vi "Measurement Logic.vi"(8 "error in":errorcluster, 11 "Measurement Configuration":T3={"Load Current in A"=0.005, "Nominal Output Voltage in V"=3.3, "Start"=4.0, "Stop"=6.0, "Step"=0.1, "Input SMU"="", "Load SMU"="", "Input DMM"="", "Load DMM"=""} {"Start" format="%#_13g"; "Nominal Output Voltage in V" format="%#_13g"; "Load Current in A" format="%#_13g"}) -> (0 "error out":errorcluster, 3 "Measurement Results":T2)   [LabVIEW 2020, in "LineRegulation.lvlib"]
uses:
  LineRegulation.lvlib
  Measurement Configuration.ctl
  Measurement Results.ctl
  Reusables/TestResults.ctl
  Reusables/TestInputs.ctl
  Reusables/Advanced Settings.ctl
  Reusables/Prepare Fn Configurations.ctl
  Reusables/Load Output Function.ctl
  Reusables/Stimulus And Measure.ctl
  67fd4621-6b8d-4ac9-96cc-a6754edf287a.vi
panel:
  out "Test Results":T1
  out "Line Regulation":cluster{"Iload (mA)":dbl[], "Vout (V)":dbl[]}(graph)
  out "Line Regulation (%)":dbl format="%#.3g"
  out "Line Regulation (%/V)":dbl format="%#.3g"
  # "Below outputs could be used to debug or verify when we run this vi as standalone"
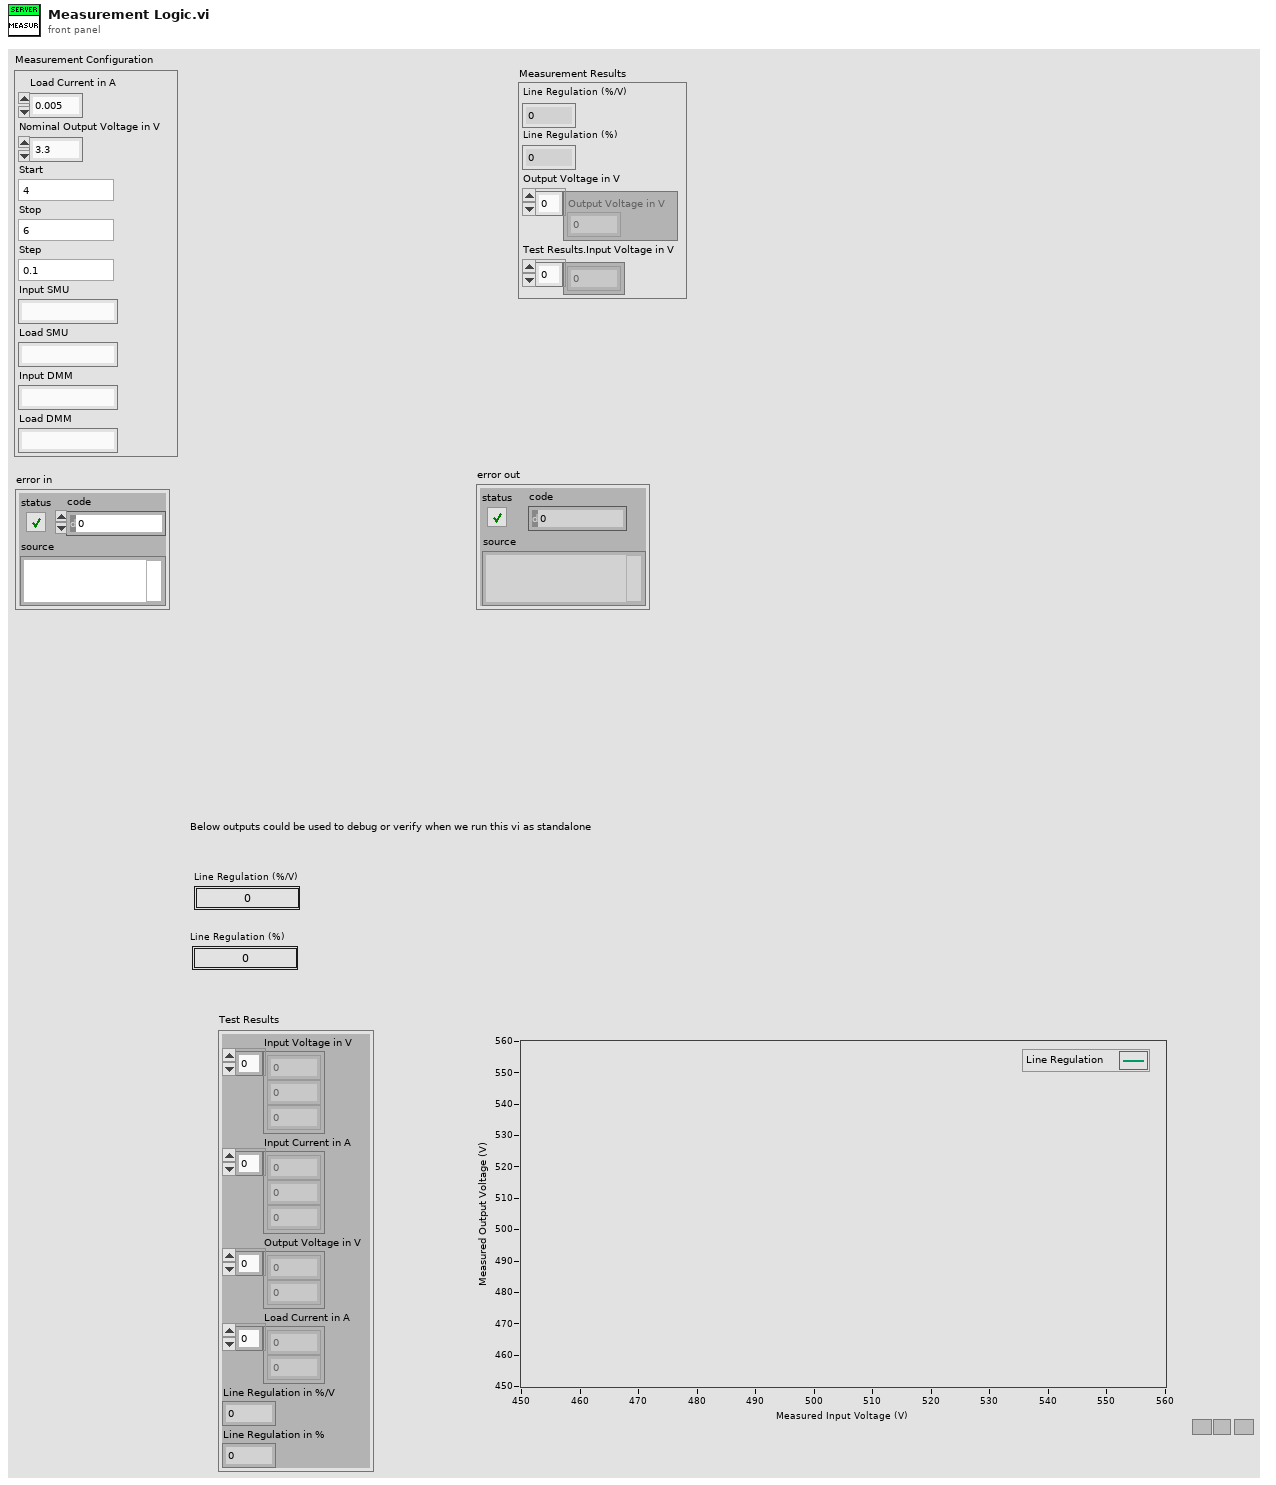
[diagram p1: front panel]
types:
  T1 = typedef "LineRegulation.lvlib/TestResults.ctl" = cluster{"Input Voltage in V":dbl[], "Input Current in A":dbl[], "Output Voltage in V":dbl[], "Load Current in A":dbl[], "Line Regulation in %/V":dbl, "Line Regulation in %":dbl}
  T2 = typedef "LineRegulation.lvlib/Measurement Results.ctl" = cluster{"Line Regulation (%/V)":dbl, "Line Regulation (%)":dbl, "Output Voltage in V":dbl[], "Test Results.Input Voltage in V":dbl[]}
  T3 = typedef "LineRegulation.lvlib/Measurement Configuration.ctl" = cluster{"Load Current in A":dbl, "Nominal Output Voltage in V":dbl, "Start":dbl, "Stop":dbl, "Step":dbl, "Input SMU":string, "Load SMU":string, "Input DMM":string, "Load DMM":string}
  T4 = typedef "LineRegulation.lvlib/TestInputs.ctl" = cluster{"Load Current in A":dbl, "Input Voltage in V":dbl[], "Nominal Output Voltage in V":dbl, "Advance Setting":T5}
  T5 = typedef "Advanced Settings.ctl" = cluster{"Prepare":T6, "Stimulus And Measure":T8}
  T6 = typedef "Prepare Fn Configurations.ctl" = cluster{"Load SMU Output Function":T7}
  T7 = typedef "Load Output Function.ctl" = enum16{"VoltageSource", "CurrentSource"}
  T8 = typedef "Stimulus And Measure.ctl" = cluster{"Loop Delay in milliSecond":u32}
  T9 = cluster{"Test Inputs":T4, "Test Results":T1, "Test Results[][]":string[][], "SMU V":refnum<k15>, "Input DMM":refnum<k15>, "Load DMM":refnum<k15>, "SMU I":refnum<k15>}
  T10 = cluster{"Input Voltage in V":dbl[], "Output Voltage in V":dbl[]}
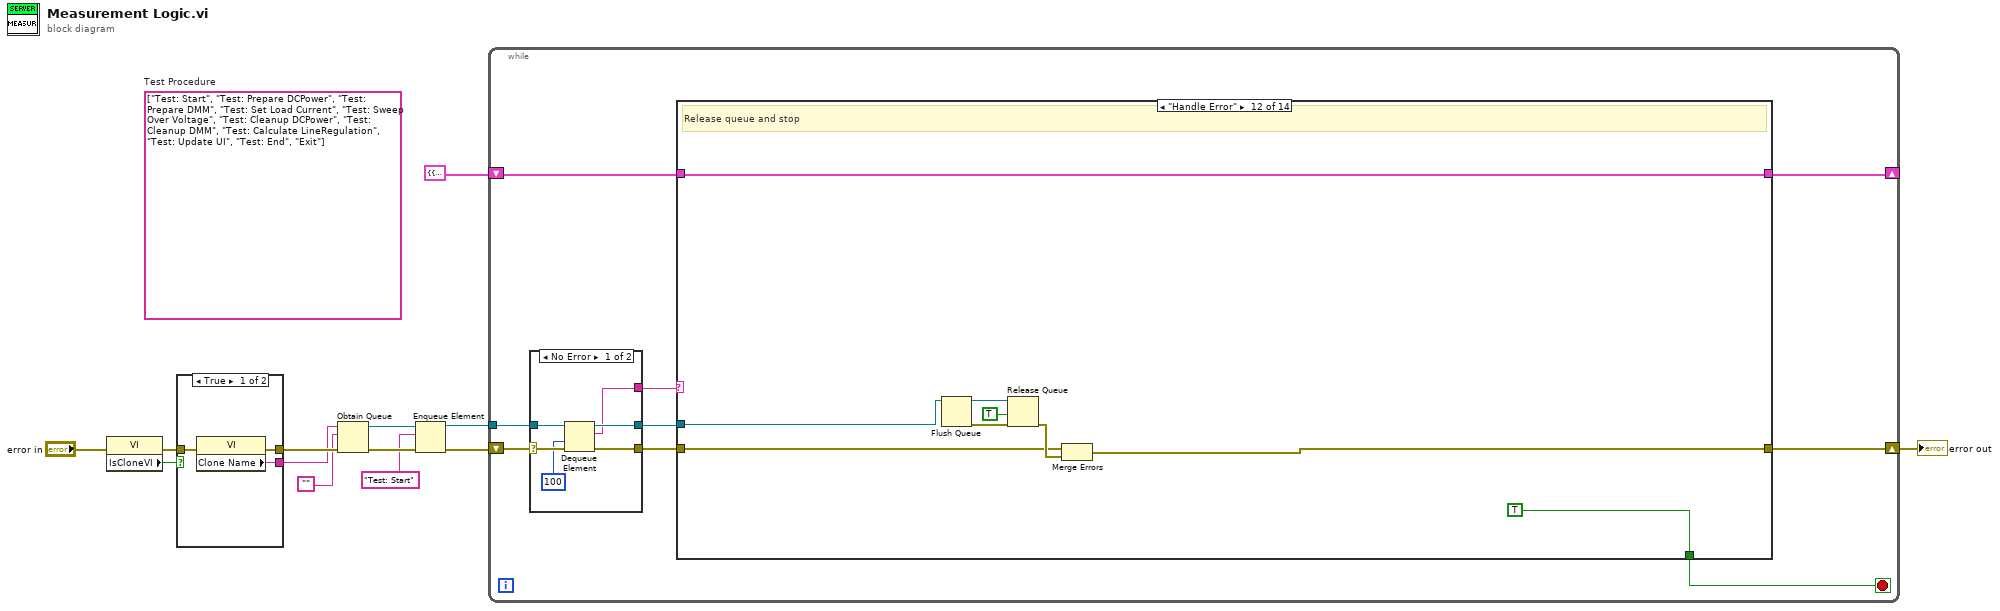
[diagram p0: block diagram]
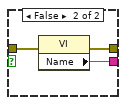
[diagram p2: hidden frame]
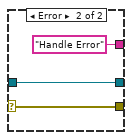
[diagram p3: hidden frame]
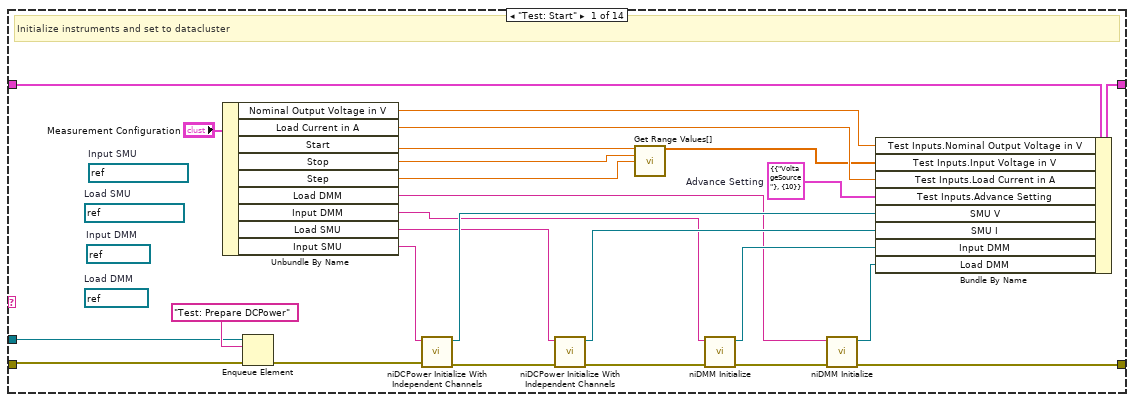
[diagram p4: hidden frame]
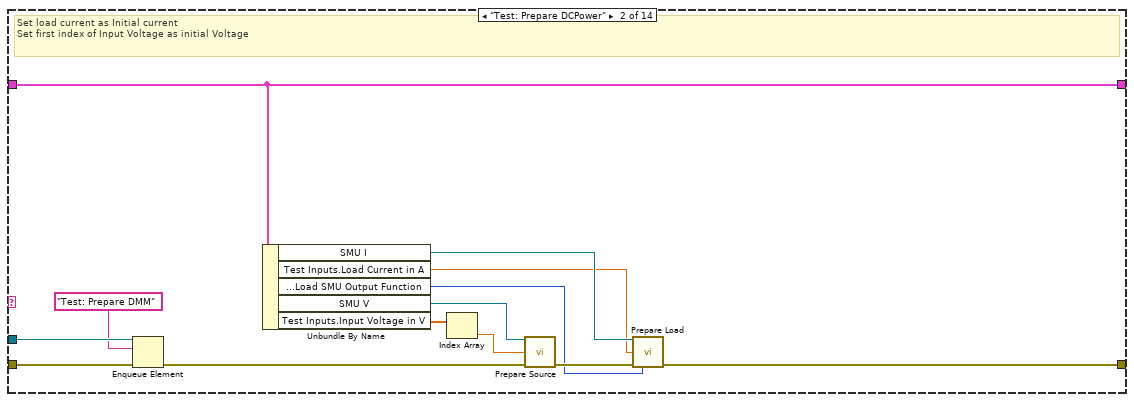
[diagram p5: hidden frame]
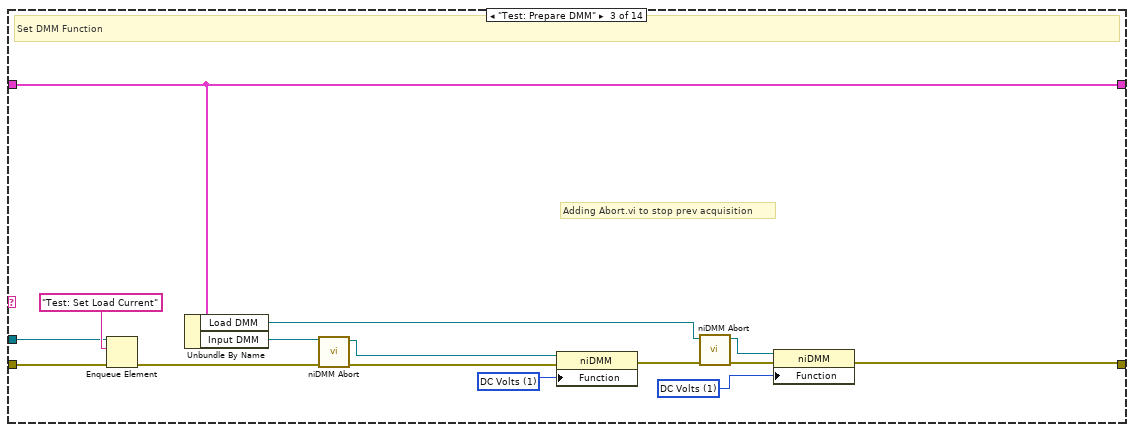
[diagram p6: hidden frame]
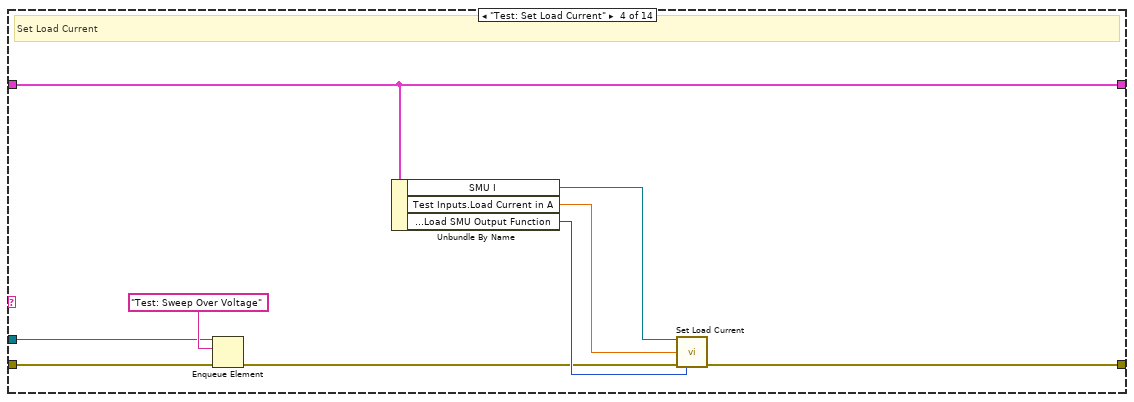
[diagram p7: hidden frame]
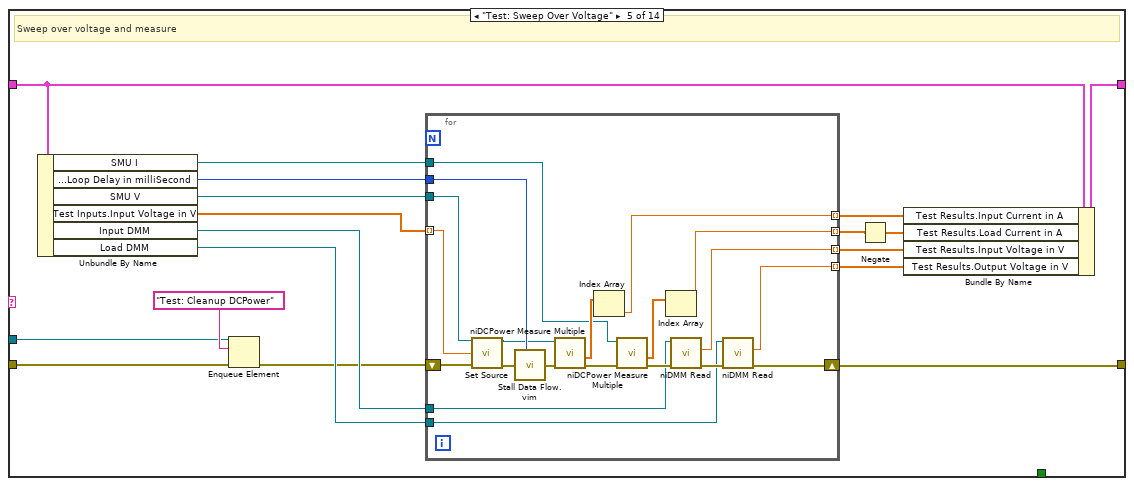
[diagram p8: hidden frame]
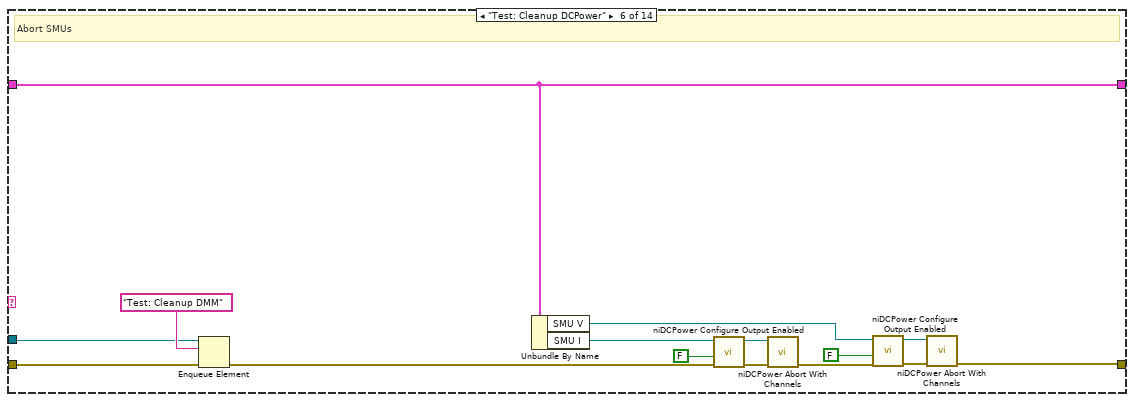
[diagram p9: hidden frame]
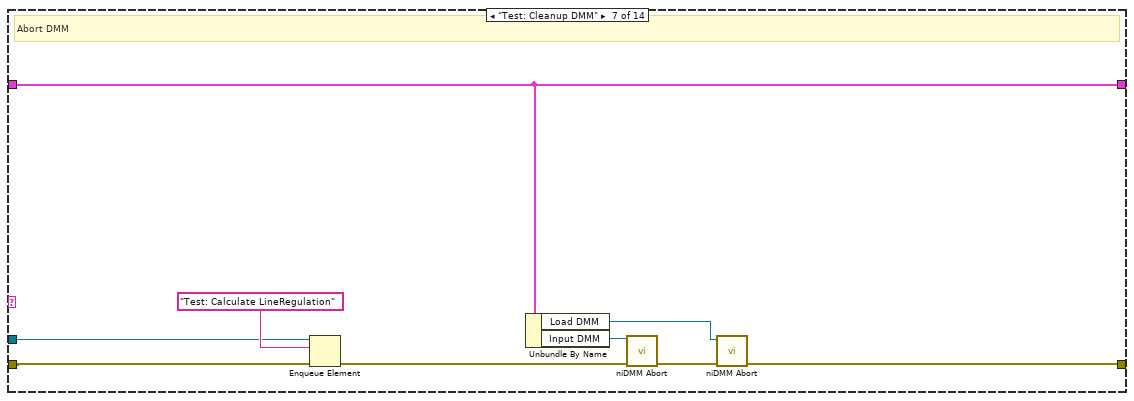
[diagram p10: hidden frame]
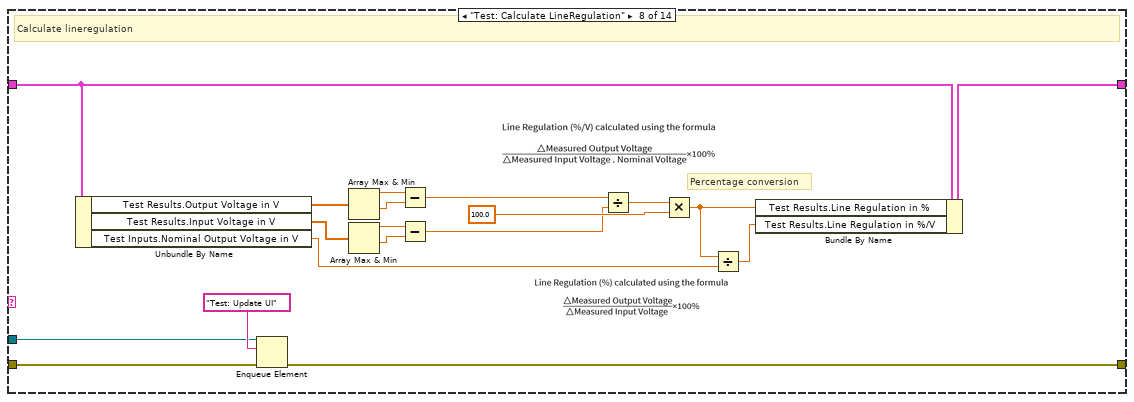
[diagram p11: hidden frame]
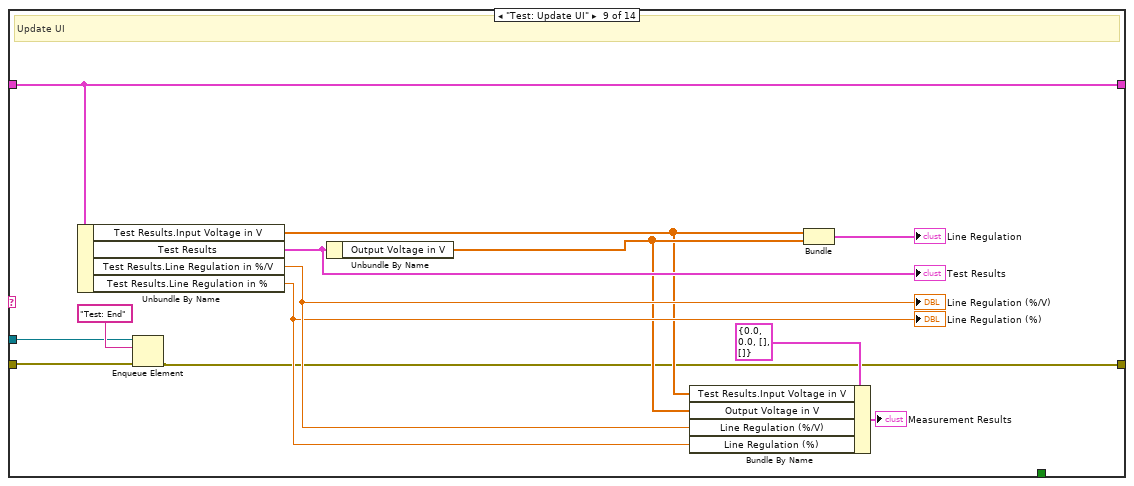
[diagram p12: hidden frame]
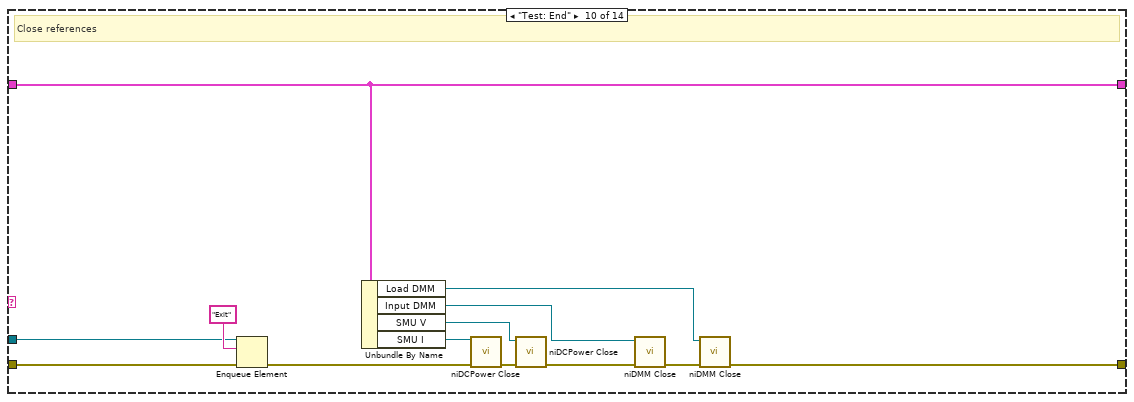
[diagram p13: hidden frame]
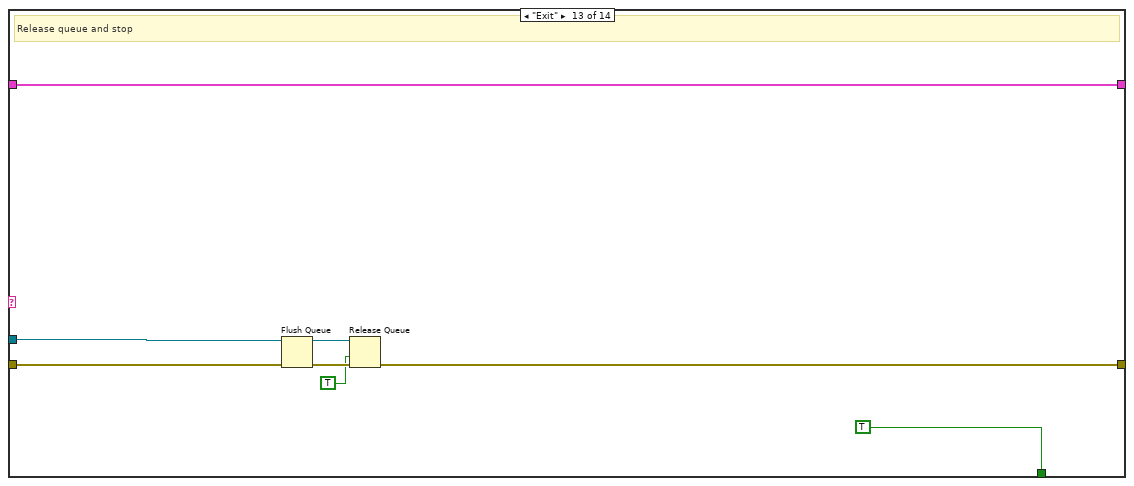
[diagram p15: hidden frame]
diagram:
  (unwired) string[] ["Test: Start", "Test: Prepare DCPower", "Test: Prepare DMM", "Test: Set Load Current", "Test: Sweep Over Voltage", "Test: Cleanup DCPower", "Test: Cleanup DMM", "Test: Calculate LineRegulation", "Test: Update UI", "Test: End", "Exit"]  # Test Procedure
  n1 = property class="VI"(error in="error in") -> (error out=w4:errorcluster, "IsCloneVI"=w5:bool)  [unwired: 1 in, 1 out]
  n2 = case shown="True" w5 {
    tunnel: [w16 w19] -> w11
    tunnel: [w15 w18] -> w10
    tunnel: w4 -> [w14 w17]
    frame True {
      n3 = property class="VI"(error in=w14) -> (error out=w16:errorcluster, "Clone Name"=w15:string)  [unwired: 1 in, 1 out]
    }
    frame False {
      n4 = property class="VI"(error in=w17) -> (error out=w19:errorcluster, "Name"=w18:string)  [unwired: 1 in, 1 out]
    }
  }
  n5 = Obtain Queue(name (unnamed)=w10, element data type="", error in (no error)=w11) -> (queue out=w8:refnum<queue>, error out=w9:errorcluster)  [unwired: 2 in, 1 out]
  n6 = Enqueue Element(queue=w8, element="Test: Start", error in (no error)=w9) -> (queue out=w1:refnum<queue>, error out=w3:errorcluster)  [unwired: 1 in, 1 out]
  n7 = while {
    shift-right: [w28] -> w12
    shift-left: w3 -> [w24]
    shift-right: [w26] -> _
    shift-left: T9 {"Test Inputs"={"Load Current in A"=0.0, "Input Voltage in V"=[], "Nominal Output Voltage in V"=0.0, "Advance Setting"={"Prepare"={"Load SMU Output Function"=enum."VoltageSource"}, "Stimulus And Measure"={"Loop Delay in milliSecond"=1}}}, "Test Results"={"Input Voltage in V"=[], "Input Current in A"=[], "Output Voltage in V"=[], "Load Current in A"=[], "Line Regulation in %/V"=0.0, "Line Regulation in %"=0.0}, "Test Results[][]"=[], "SMU V"="", "Input DMM"="", "Load DMM"="", "SMU I"=""} -> [w27]
    tunnel: w1 -> [w20]
    stop <- w25 stop-if-true
    n8 = case shown="No Error" w24 {
      selector: w24 -> [w34 w37]
      tunnel: [w33 w37] -> w21
      tunnel: w20 -> [w32 w36]
      tunnel: [w31 w36] -> w23
      tunnel: [w30 "Handle Error"] -> w22
      frame No Error {
        n9 = Dequeue Element(queue=w32, timeout in ms (-1)=100, error in (no error)=w34) -> (queue out=w31:refnum<queue>, element=w30:string, error out=w33:errorcluster)  [unwired: 1 out]
      }
      frame Error {
      }
    }
    n10 = case shown="\"Handle Error\"" w22 {
      tunnel: w23 -> [w41 w65 w79 w92 w101 w139 w154 w165 w184 w195 _ w212 w219 _]
      tunnel: w21 -> [w40 w66 w77 w93 w103 w140 w155 w163 w182 w196 w209 w210 w221 w227]
      tunnel: [w38 w69 w82 w96 w108 w150 w160 w164 w183 w201 w209 w217 w220 w227] -> w28
      tunnel: w27 -> [w62 w75 w88 w100 w106 w149 w162 w167 w192 w207 w208 w218 w226 w228]
      tunnel: [w63 w75 w88 w100 w107 w149 w162 w168 w192 w207 w208 w218 w226 w228] -> w26
      tunnel: [_ _ _ _ _ _ _ _ _ _ _ TRUE TRUE _] -> w25
      frame "Test: Start" {
        w54 = T5 {"Prepare"={"Load SMU Output Function"=enum."VoltageSource"}, "Stimulus And Measure"={"Loop Delay in milliSecond"=10}}  # Advance Setting
        (unwired) refnum<k15> "DPS_4145_1/3"  # Load SMU
        (unwired) refnum<k15> "DMM2"  # Load DMM
        (unwired) refnum<k15> "DMM1"  # Input DMM
        (unwired) refnum<k15> "DPS_4145_1/1"  # Input SMU
        # "Initialize instruments and set to datacluster"
        n11 = Unbundle By Name("Measurement Configuration") -> ("Nominal Output Voltage in V"=w52:dbl, "Load Current in A"=w51:dbl, "Start"=w50:dbl, "Stop"=w49:dbl, "Step"=w48:dbl, "Load DMM"=w46:string, "Input DMM"=w45:string, "Load SMU"=w44:string, "Input SMU"=w43:string)
        n12 = Enqueue Element(queue=w41, element="Test: Prepare DCPower", error in (no error)=w40) -> (error out=w39:errorcluster)  [unwired: 1 in, 2 out]
        n13 = call <instrlib>:"niDCPower Initialize With Independent Channels.vi"("error in (no error)"=w39, "resource name"=w43) -> ("error out"=w58:errorcluster, "instrument handle out"=w61:refnum<k15>)  [unwired: 8 in]
        n14 = call <instrlib>:"niDCPower Initialize With Independent Channels.vi"("error in (no error)"=w58, "resource name"=w44) -> ("error out"=w57:errorcluster, "instrument handle out"=w55:refnum<k15>)  [unwired: 8 in]
        n15 = call "Get Range Values[].vi"("Start"=w50, "Stop"=w49, "Step Size"=w48) -> ("Values[]"=w47:dbl[])  [unwired: 12 in]
        n16 = call <instrlib>:"niDMM Initialize.vi"("error in (no error)"=w57, "Instrument Descriptor"=w45) -> ("error out"=w59:errorcluster, "instrument handle out"=w56:refnum<k15>)  [unwired: 8 in]
        n17 = call <instrlib>:"niDMM Initialize.vi"("error in (no error)"=w59, "Instrument Descriptor"=w46) -> ("error out"=w38:errorcluster, "instrument handle out"=w60:refnum<k15>)  [unwired: 8 in]
        n18 = Bundle By Name(cluster=w62, "Test Inputs.Nominal Output Voltage in V"=w52, "Test Inputs.Input Voltage in V"=w47, "Test Inputs.Load Current in A"=w51, "Test Inputs.Advance Setting"=w54, "SMU V"=w61, "SMU I"=w55, "Input DMM"=w56, "Load DMM"=w60) -> (w63:T9)
      }
      frame "Test: Prepare DCPower" {
        # "Set load current as Initial current\nSet first index of Input Voltage as initial Voltage"
        n19 = Enqueue Element(queue=w65, element="Test: Prepare DMM", error in (no error)=w66) -> (error out=w67:errorcluster)  [unwired: 1 in, 2 out]
        n20 = Unbundle By Name(w75) -> ("SMU I"=w72:refnum<k15>, "Test Inputs.Load Current in A"=w71:dbl, "Test Inputs.Advance Setting.Prepare.Load SMU Output Function"=w68:T7, "SMU V"=w74:refnum<k15>, "Test Inputs.Input Voltage in V"=w76:dbl[])
        n21 = Index Array(array=w76) -> (element=w73:dbl)  [unwired: 1 in]
        n22 = call "Prepare Source.vi"("instrument handle"=w74, "Initial Voltage Level (V)"=w73, "error in (no error)"=w67) -> ("error out"=w70:errorcluster)  [unwired: 12 in]
        n23 = call "Prepare Load.vi"("instrument handle"=w72, "Load Current Level (A)"=w71, "error in (no error)"=w70, "Load Output Function"=w68) -> ("error out"=w69:errorcluster)  [unwired: 11 in]
      }
      frame "Test: Prepare DMM" {
        w84 = 1 items=["DC Volts"=1, "AC Volts"=2, "DC Current"=3, "AC Current"=4, "2-Wire Resistance"=5, "4-Wire Resistance"=101, "Frequency"=104, "Period"=105, "AC Volts DC Coupled"=1001, "Diode"=1002, "Waveform Voltage"=1003, "Waveform Current"=1004, "Capacitance"=1005, "Inductance"=1006, "Temperature"=108] ("Configuration:Function")
        w91 = 1 items=["DC Volts"=1, "AC Volts"=2, "DC Current"=3, "AC Current"=4, "2-Wire Resistance"=5, "4-Wire Resistance"=101, "Frequency"=104, "Period"=105, "AC Volts DC Coupled"=1001, "Diode"=1002, "Waveform Voltage"=1003, "Waveform Current"=1004, "Capacitance"=1005, "Inductance"=1006, "Temperature"=108] ("Configuration:Function")
        # "Adding Abort.vi to stop prev acquisition"
        # "Set DMM Function"
        n24 = Enqueue Element(queue=w79, element="Test: Set Load Current", error in (no error)=w77) -> (error out=w78:errorcluster)  [unwired: 1 in, 2 out]
        n25 = Unbundle By Name(w88) -> ("Load DMM"=w81:refnum<k15>, "Input DMM"=w87:refnum<k15>)
        n26 = call <instrlib>:"niDMM Abort.vi"("error in (no error)"=w78, "instrument handle"=w87) -> ("error out"=w90:errorcluster, "instrument handle out"=w89:refnum<k15>)  [unwired: 8 in]
        n27 = property class="niDMM"(reference=w89, error in=w90, "Function"=w91) -> (error out=w83:errorcluster)  [unwired: 1 out]
        n28 = call <instrlib>:"niDMM Abort.vi"("error in (no error)"=w83, "instrument handle"=w81) -> ("error out"=w85:errorcluster, "instrument handle out"=w86:refnum<k15>)  [unwired: 8 in]
        n29 = property class="niDMM"(reference=w86, error in=w85, "Function"=w84) -> (error out=w82:errorcluster)  [unwired: 1 out]
      }
      frame "Test: Set Load Current" {
        # "Set Load Current"
        n30 = Enqueue Element(queue=w92, element="Test: Sweep Over Voltage", error in (no error)=w93) -> (error out=w94:errorcluster)  [unwired: 1 in, 2 out]
        n31 = Unbundle By Name(w100) -> ("SMU I"=w99:refnum<k15>, "Test Inputs.Load Current in A"=w98:dbl, "Test Inputs.Advance Setting.Prepare.Load SMU Output Function"=w97:T7)
        n32 = call "Set Load Current.vi"("instrument handle in"=w99, "current level"=w98, "error in (no error)"=w94, "OutputFunction"=w97) -> ("error out"=w96:errorcluster)  [unwired: 10 in, 1 out]
      }
      frame "Test: Sweep Over Voltage" {
        # "Sweep over voltage and measure"
        n33 = Unbundle By Name(w106) -> ("SMU I"=w105:refnum<k15>, "Test Inputs.Advance Setting.Stimulus And Measure.Loop Delay in milliSecond"=w116:u32, "SMU V"=w118:refnum<k15>, "Test Inputs.Input Voltage in V"=w117:dbl[], "Input DMM"=w115:refnum<k15>, "Load DMM"=w114:refnum<k15>)
        n34 = Enqueue Element(queue=w101, element="Test: Cleanup DCPower", error in (no error)=w103) -> (error out=w102:errorcluster)  [unwired: 1 in, 2 out]
        n35 = for {
          tunnel: w118 -> [w137]
          tunnel: w117 -> [w136] mode=indexing
          tunnel: w116 -> [w134]
          tunnel: w115 -> [w127]
          tunnel: w114 -> [w126]
          tunnel: [w125] -> w112 mode=indexing
          tunnel: [w124] -> w111 mode=indexing
          tunnel: [w123] -> w110 mode=indexing
          tunnel: [w122] -> w109 mode=indexing
          shift-right: [w121] -> w108
          shift-left: w102 -> [w138]
          tunnel: w105 -> [w119]
          n36 = call "Set Source.vi"("instrument handle in"=w137, "Vin in V"=w136, "error in (no error)"=w138) -> ("instrument handle out"=w120:refnum<k15>, "error out"=w135:errorcluster)  [unwired: 11 in]
          n37 = call "Stall Data Flow.vim"("value in"=w135, "milliseconds to wait"=w134) -> ("value out"=w128:errorcluster)  [unwired: 1 out]
          n38 = call <instrlib>:"niDCPower Measure Multiple.vi"("error in (no error)"=w128, "instrument handle"=w120) -> ("error out"=w130:errorcluster, "current measurements"=w133:dbl[])  [unwired: 6 in, 2 out]
          n39 = Index Array(array=w133) -> (element=w125:dbl)  [unwired: 1 in]
          n40 = call <instrlib>:"niDCPower Measure Multiple.vi"("error in (no error)"=w130, "instrument handle"=w119) -> ("error out"=w129:errorcluster, "current measurements"=w131:dbl[])  [unwired: 6 in, 2 out]
          n41 = Index Array(array=w131) -> (element=w124:dbl)  [unwired: 1 in]
          n42 = call <instrlib>:"niDMM Read.vi"("error in (no error)"=w129, "instrument handle"=w127) -> ("error out"=w132:errorcluster, "Measurement"=w123:dbl)  [unwired: 7 in, 1 out]
          n43 = call <instrlib>:"niDMM Read.vi"("error in (no error)"=w132, "instrument handle"=w126) -> ("error out"=w121:errorcluster, "Measurement"=w122:dbl)  [unwired: 7 in, 1 out]
        }
        n44 = Negate(x=w111) -> (-x=w113:dbl[])
        n45 = Bundle By Name(cluster=w106, "Test Results.Input Current in A"=w112, "Test Results.Load Current in A"=w113, "Test Results.Input Voltage in V"=w110, "Test Results.Output Voltage in V"=w109) -> (w107:T9)
      }
      frame "Test: Cleanup DCPower" {
        # "Abort SMUs"
        n46 = Enqueue Element(queue=w139, element="Test: Cleanup DMM", error in (no error)=w140) -> (error out=w141:errorcluster)  [unwired: 1 in, 2 out]
        n47 = Unbundle By Name(w149) -> ("SMU V"=w148:refnum<k15>, "SMU I"=w143:refnum<k15>)
        n48 = call <instrlib>:"niDCPower Configure Output Enabled.vi"("error in (no error)"=w141, "output enabled"=FALSE, "instrument handle"=w143) -> ("error out"=w144:errorcluster, "instrument handle out"=w147:refnum<k15>)  [unwired: 7 in]
        n49 = call <instrlib>:"niDCPower Abort With Channels.vi"("error in (no error)"=w144, "instrument handle"=w147) -> ("error out"=w145:errorcluster)  [unwired: 8 in, 1 out]
        n50 = call <instrlib>:"niDCPower Configure Output Enabled.vi"("error in (no error)"=w145, "output enabled"=FALSE, "instrument handle"=w148) -> ("error out"=w152:errorcluster, "instrument handle out"=w151:refnum<k15>)  [unwired: 7 in]
        n51 = call <instrlib>:"niDCPower Abort With Channels.vi"("error in (no error)"=w152, "instrument handle"=w151) -> ("error out"=w150:errorcluster)  [unwired: 8 in, 1 out]
      }
      frame "Test: Cleanup DMM" {
        # "Abort DMM"
        n52 = Enqueue Element(queue=w154, element="Test: Calculate LineRegulation", error in (no error)=w155) -> (error out=w156:errorcluster)  [unwired: 1 in, 2 out]
        n53 = Unbundle By Name(w162) -> ("Load DMM"=w159:refnum<k15>, "Input DMM"=w158:refnum<k15>)
        n54 = call <instrlib>:"niDMM Abort.vi"("error in (no error)"=w156, "instrument handle"=w158) -> ("error out"=w161:errorcluster)  [unwired: 8 in, 1 out]
        n55 = call <instrlib>:"niDMM Abort.vi"("error in (no error)"=w161, "instrument handle"=w159) -> ("error out"=w160:errorcluster)  [unwired: 8 in, 1 out]
      }
      frame "Test: Calculate LineRegulation" {
        # "Percentage conversion"
        # "Calculate lineregulation"
        n56 = Unbundle By Name(w167) -> ("Test Results.Output Voltage in V"=w179:dbl[], "Test Results.Input Voltage in V"=w174:dbl[], "Test Inputs.Nominal Output Voltage in V"=w170:dbl)
        n57 = Enqueue Element(queue=w165, element="Test: Update UI", error in (no error)=w163) -> (error out=w164:errorcluster)  [unwired: 1 in, 2 out]
        n58 = Array Max & Min(array=w179) -> (max value=w181:dbl, min value=w177:dbl)  [unwired: 2 out]
        n59 = Array Max & Min(array=w174) -> (max value=w175:dbl, min value=w176:dbl)  [unwired: 2 out]
        n60 = Subtract(x=w181, y=w177) -> (x-y=w178:dbl)
        n61 = Subtract(x=w175, y=w176) -> (x-y=w173:dbl)
        n62 = Divide(x=w178, y=w173) -> (x/y=w172:dbl)
        n63 = Multiply(x=w172, y=100.0) -> (x*y=w171:dbl)
        n64 = Divide(x=w171, y=w170) -> (x/y=w169:dbl)
        n65 = Bundle By Name(cluster=w167, "Test Results.Line Regulation in %"=w171, "Test Results.Line Regulation in %/V"=w169) -> (w168:T9)
      }
      frame "Test: Update UI" {
        # "Update UI"
        n66 = Unbundle By Name(w192) -> ("Test Results.Input Voltage in V"=w186:dbl[], "Test Results"=w193:T1, "Test Results.Line Regulation in %/V"=w189:dbl, "Test Results.Line Regulation in %"=w188:dbl)
        "Line Regulation (%/V)" <- w189
        "Line Regulation (%)" <- w188
        "Test Results" <- w193
        n67 = Enqueue Element(queue=w184, element="Test: End", error in (no error)=w182) -> (error out=w183:errorcluster)  [unwired: 1 in, 2 out]
        n68 = Unbundle By Name(w193) -> ("Output Voltage in V"=w187:dbl[])
        n69 = Bundle By Name(cluster=T2 {"Line Regulation (%/V)"=0.0, "Line Regulation (%)"=0.0, "Output Voltage in V"=[], "Test Results.Input Voltage in V"=[]} ("Measurement Results"), "Test Results.Input Voltage in V"=w186, "Output Voltage in V"=w187, "Line Regulation (%/V)"=w189, "Line Regulation (%)"=w188) -> (→"Measurement Results":T2)
        n70 = Bundle("Input Voltage in V"=w186, "Output Voltage in V"=w187) -> (→"Line Regulation":T10)  [unwired: 1 in]
      }
      frame "Test: End" {
        # "Close references"
        n71 = Enqueue Element(queue=w195, element="Exit", error in (no error)=w196) -> (error out=w197:errorcluster)  [unwired: 1 in, 2 out]
        n72 = Unbundle By Name(w207) -> ("Load DMM"=w202:refnum<k15>, "Input DMM"=w203:refnum<k15>, "SMU V"=w206:refnum<k15>, "SMU I"=w200:refnum<k15>)
        n73 = call <instrlib>:"niDCPower Close.vi"("error in (no error)"=w197, "instrument handle"=w200) -> ("error out"=w199:errorcluster)  [unwired: 9 in]
        n74 = call <instrlib>:"niDCPower Close.vi"("error in (no error)"=w199, "instrument handle"=w206) -> ("error out"=w205:errorcluster)  [unwired: 9 in]
        n75 = call <instrlib>:"niDMM Close.vi"("error in (no error)"=w205, "instrument handle"=w203) -> ("error out"=w204:errorcluster)  [unwired: 9 in]
        n76 = call <instrlib>:"niDMM Close.vi"("error in (no error)"=w204, "instrument handle"=w202) -> ("error out"=w201:errorcluster)  [unwired: 9 in]
      }
      frame "----Misc------" {
      }
      frame "Handle Error" {
        # "Release queue and stop"
        n77 = Flush Queue(queue=w212) -> (queue out=w215:refnum<queue>, error out=w214:errorcluster)  [unwired: 1 in, 1 out]
        n78 = Release Queue(queue=w215, force destroy? (F)=TRUE, error in (no error)=w214) -> (error out=w211:errorcluster)  [unwired: 2 out]
        n79 = Merge Errors(w210, w211) -> (w217:errorcluster)
      }
      frame "Exit" {
        # "Release queue and stop"
        n80 = Flush Queue(queue=w219, error in (no error)=w221) -> (queue out=w224:refnum<queue>, error out=w223:errorcluster)  [unwired: 1 out]
        n81 = Release Queue(queue=w224, force destroy? (F)=TRUE, error in (no error)=w223) -> (error out=w220:errorcluster)  [unwired: 2 out]
      }
      frame "", Default {
        # "Do nothing"
      }
    }
  }
  "error out" <- w12
